vi "Report_Preview_Error.vi"(8 "error in (no error)":errorcluster, 11 "IB_Source in":refnum<class "IB_Source.lvclass">) -> (0 "error out":errorcluster, 3 "IB_Source out":refnum<class "IB_Source.lvclass">)   [LabVIEW 2020, in "IB_Source.lvclass"]
uses:
  <vilib>/AppBuilder/IB_Classes/Source/IB_Source.lvclass
  <vilib>/AppBuilder/IB_Classes/Source/IB_Source.lvclass/IB_Source.ctl
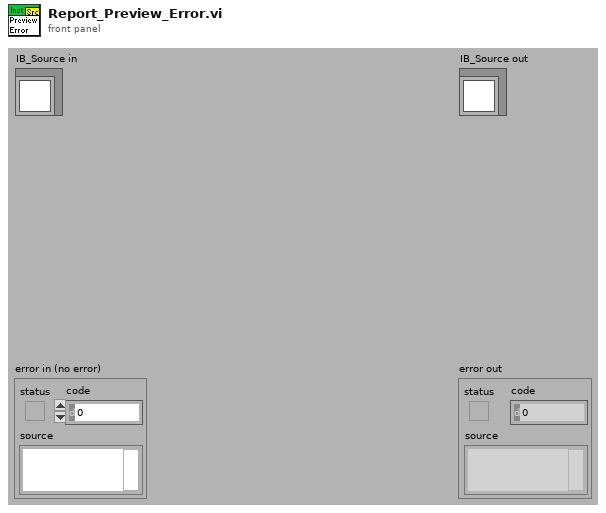
[diagram p1: front panel]
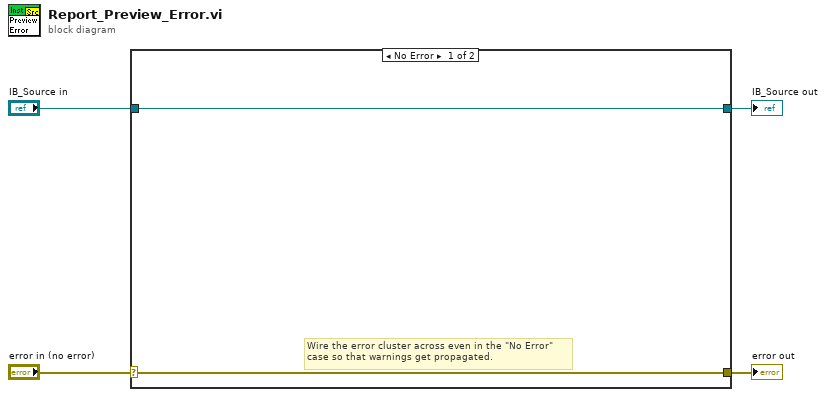
[diagram p0: block diagram]
diagram:
  n1 = case shown="No Error" "error in (no error)" {
    selector: "error in (no error)" -> [w5 w8]
    tunnel: [w5 w8] -> w3
    tunnel: [w6 w7] -> w1
    tunnel: "IB_Source in" -> [w6 w7]
    frame No Error {
      # "Wire the error cluster across even in the \"No Error\"\ncase so that warnings get propagated."
    }
    frame Error {
    }
  }
  "error out" <- w3
  "IB_Source out" <- w1
